vi "mapa.vi"() -> ()   [LabVIEW 2021]
panel:
  in  "stop":bool
  out "concatenated string 2":string
  in  "Zoom":i32
  in  "Longitude":dbl format="%#_10g"
  in  "Latitude":dbl format="%#_8g"
  in  "WebBrowser":refnum<k7>(container)
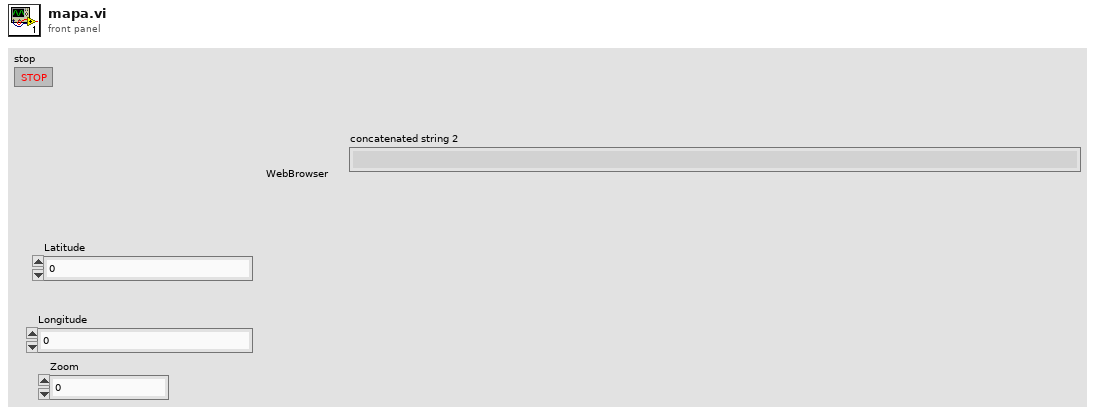
[diagram p1: front panel]
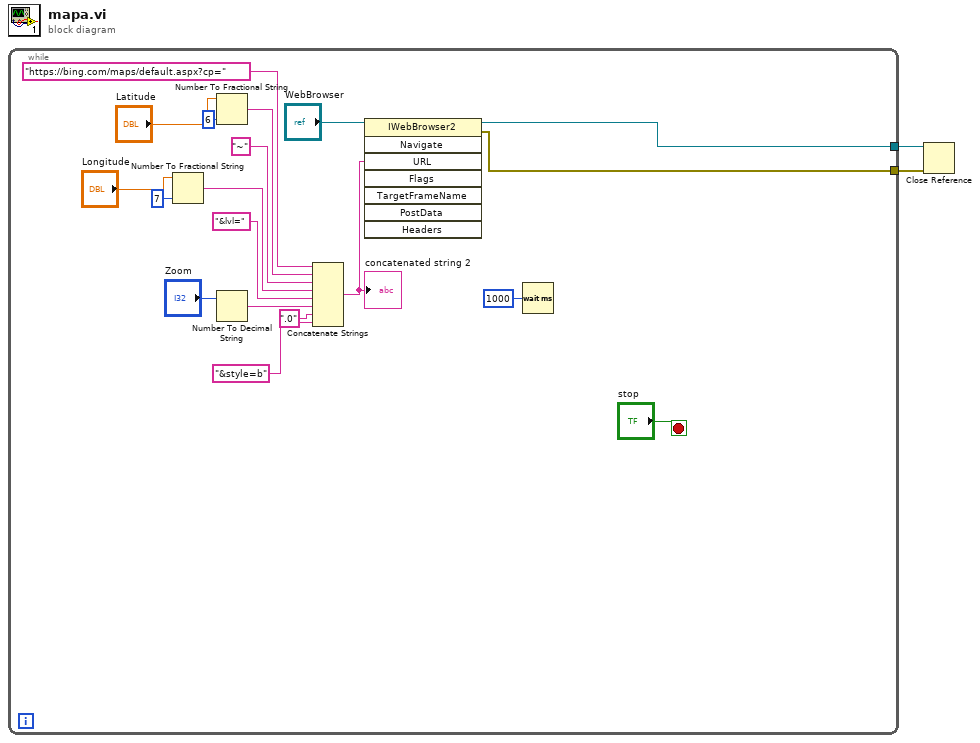
[diagram p0: block diagram]
diagram:
  n1 = while {
    tunnel: [w4] -> w2
    tunnel: [w3] -> w1
    stop <- "stop" stop-if-true
    n2 = Number To Fractional String(number="Longitude", precision (6)=i16 7) -> (F-format string=w16:string)  [unwired: 2 in]
    n3 = Number To Fractional String(number="Latitude", precision (6)=i16 6) -> (F-format string=w19:string)  [unwired: 2 in]
    n4 = Number To Decimal String(number="Zoom") -> (decimal integer string=w13:string)  [unwired: 1 in]
    n5 = Concatenate Strings("https://bing.com/maps/default.aspx?cp=", w19, "~", w16, "&lvl=", w13, ".0" ("string"), "&style=b" ("string")) -> (w12:string)
    "concatenated string 2" <- w12
    n6 = invoke class="IWebBrowser2" method="Navigate"(reference="WebBrowser", "URL"=w12) -> (reference out=w3:refnum<k7>, error out=w4:errorcluster)  [unwired: 6 in, 6 out]
    n7 = Wait (ms)(milliseconds to wait=u32 1000) -> ()  [unwired: 1 out]
  }
  n8 = Close Reference(reference=w1, error in (no error)=w2) -> ()  [unwired: 1 out]
